vi "niRFSysCalReader Add CalPathInfo.vi"(8 "error in":errorcluster, 10 "CalPath Info":T1, 11 "niRFSysCalReader Handle":T2) -> (0 "error out":errorcluster, 3 "niRFSysCalReader Handle out":T2)   [LabVIEW 2017, in "niRFSysCalReader.lvlib"]
uses:
  niRFSysCalReader.lvlib
  INCLUDES/niRFSysCalReader Handle.ctl
  INCLUDES/niRFSysCalReader CalPath Info.ctl
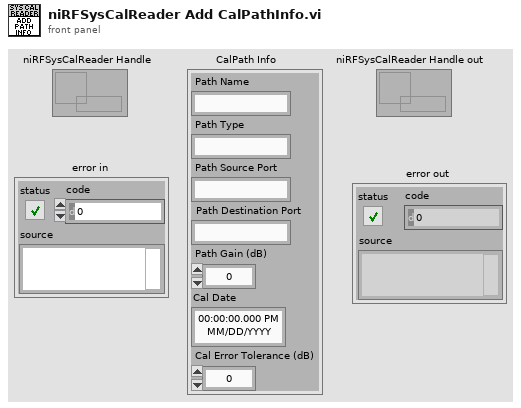
[diagram p1: front panel]
types:
  T1 = typedef "niRFSysCalReader.lvlib/niRFSysCalReader CalPath Info.ctl" = cluster{"Path Name":string, "Path Type":string, "Path Source Port":string, "Path Destination Port":string, "Path Gain (dB)":dbl, "Cal Date":timestamp, "Cal Error Tolerance (dB)":dbl}
  T2 = typedef "niRFSysCalReader.lvlib/niRFSysCalReader Handle.ctl" = refnum<data-value>
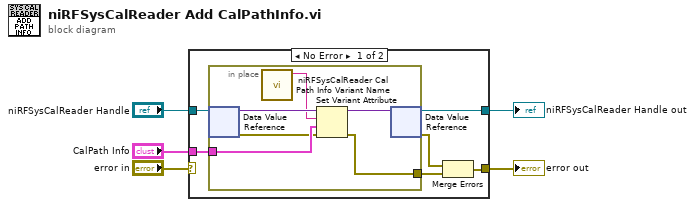
[diagram p0: block diagram]
diagram:
  n1 = case shown="No Error" "error in" {
    selector: "error in" -> [_ w19]
    tunnel: [w11 w18] -> w5
    tunnel: "niRFSysCalReader Handle" -> [w10 w18]
    tunnel: [w9 w19] -> w2
    tunnel: "CalPath Info" -> [w6 _]
    frame No Error {
      n2 = in-place {
        in-place-border: [w13] -> w7
        in-place-border: w6 -> [w14]
        n3 = in-place-dvr #1(w10) -> (w17:variant, w12:errorcluster)
        n4 = call "niRFSysCalReader Cal Path Info Variant Name.vi"() -> ("Cal Path Info Name"=w16:string)  [unwired: 11 in]
        n5 = Set Variant Attribute(Variant=w17, name=w16, value=w14, error in=w12) -> (Variant out=w15:variant, error out=w13:errorcluster)  [unwired: 1 out]
        n6 = in-place-dvr #1(w15) -> (w11:T2, w8:errorcluster)
      }
      n7 = Merge Errors(w8, w7) -> (w9:errorcluster)
    }
    frame Error {
    }
  }
  "niRFSysCalReader Handle out" <- w5
  "error out" <- w2
